vi "meTEC_Re-Init after Error (Monitoring Loop).vi"(8 "error in (no error)":errorcluster) -> (0 "error out":errorcluster)   [LabVIEW 2019]
panel:
  # "--- Outputs ---"
  # "--- Inputs ---"
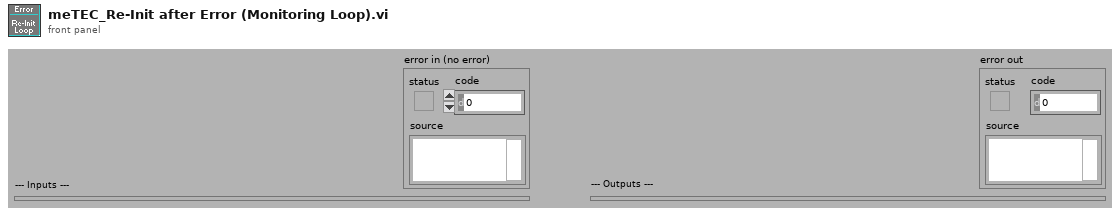
[diagram p1: front panel]
types:
  T1 = typedef "FGV_TE Controller.ctl" = cluster{"SVs":cluster{"Unused":dbl}, "PVs":cluster{"FW & HW Versions":cluster{"Device Type [I32]":i32, "Device Type [String]":string, "Firmware Version [I32]":i32, "Firmware Version [String]":string, "Hardware Version [I32]":i32, "Hardware Version [String]":string, "Serial No.":i32}, "TEC Configuration":T2, "Object Target Temperature Source_CH1":u8, "Object Target Temperature Source_CH2":u8}, "Front Panel References":T3}
  T2 = typedef "meTEC_Configuration.ctl" = cluster{"VISA resource name":refnum<visa-resource-name>, "Device Address":u16}
  T3 = typedef "FGV_Front Panel References.ctl" = cluster{"Main Loop Queue":refnum<queue>, "meTEC_Device Type":refnum<vi>, "meTEC_Serial No.":refnum<vi>, "meTEC_Hardware Version":refnum<vi>, "meTEC_Firmware Version":refnum<vi>, "meTEC_CH1_Object Target Temperature (ID 3000 / 50012) [°C]":refnum<vi>, "meTEC_CH1_Live Set Current (ID 50001) [A]":refnum<vi>, "meTEC_CH1_Live Set Voltage (ID 50002) [V]":refnum<vi>, "meTEC_CH1_Live Enable (ID 50000)":refnum<vi>, "meTEC_CH1_Input Selection (ID 2000)":refnum<vi>, "meTEC_CH1_Object Target Temp. Source Sel. (ID 50011)":refnum<vi>, "meTEC_CH2_Object Target Temperature (ID 3000 / 50012) [°C]":refnum<vi>, "meTEC_CH2_Live Set Current (ID 50001) [A]":refnum<vi>, "meTEC_CH2_Live Set Voltage (ID 50002) [V]":refnum<vi>, "meTEC_CH2_Live Enable (ID 50000)":refnum<vi>, "meTEC_CH2_Input Selection (ID 2000)":refnum<vi>, "meTEC_CH2_Object Target Temp. Source Sel. (ID 50011)":refnum<vi>, "meTEC_CH2_Object Temperature [°C]":refnum<vi>, "meTEC_CH2_Sink Temperature [°C]":refnum<vi>, "meTEC_CH2_Act. Output Current [A]":refnum<vi>, "meTEC_CH2_Act. Output Voltage [V]":refnum<vi>, "meTEC_CH2_Temperature Stability":refnum<vi>, "Monitor Chart_CH2":refnum<vi>, "meTEC_Initialize Device":refnum<vi>}
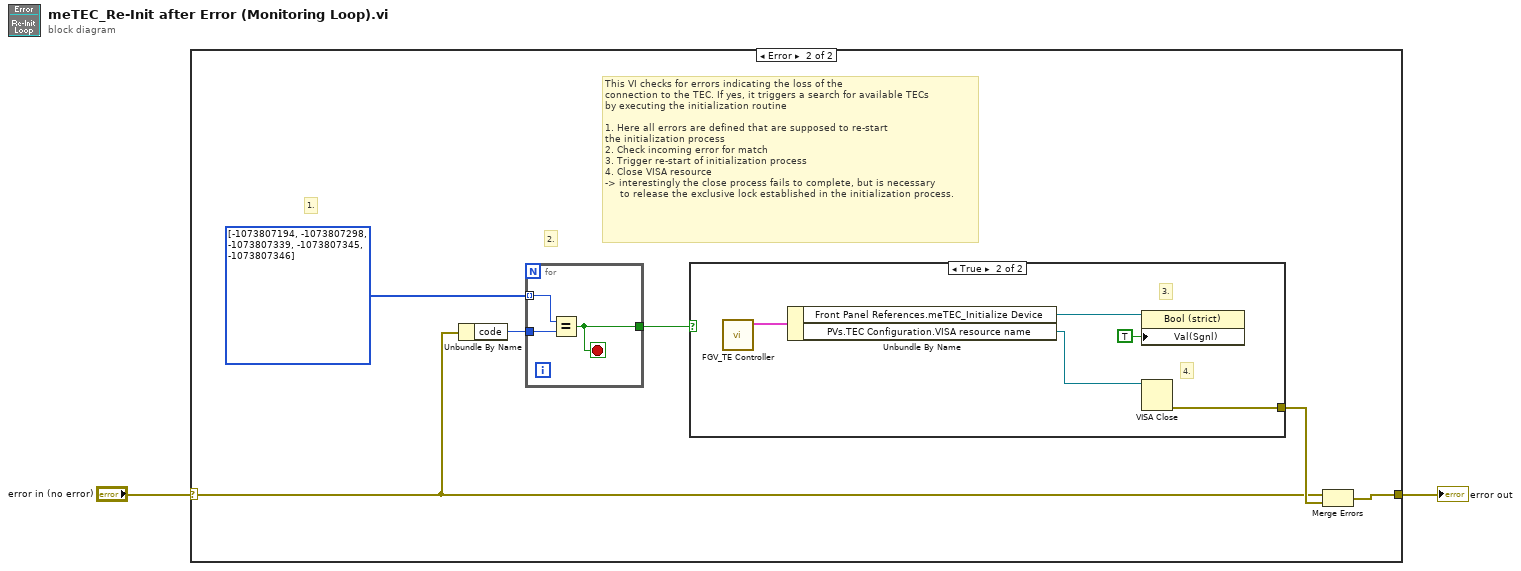
[diagram p0: block diagram]
diagram:
  n1 = case shown="Error" "error in (no error)" {
    selector: "error in (no error)" -> [w3 w5]
    tunnel: [w3 w4] -> w1
    frame No Error {
    }
    frame Error {
      # "This VI checks for errors indicating the loss of the\nconnection to the TEC. If yes, it triggers a search for available TECs\nby executing the initialization routine\n\n1. Here all errors are defined that are supposed to re-start \nthe initialization process\n2. Check incoming error for match\n3. Trigger re-start of initialization process\n4. Close VISA resource\n-> interestingly the close process fails to complete, but is necessary\n     to release the exclusive lock established in the initialization process."
      # "2."
      # "1."
      n2 = Unbundle By Name(w5) -> ("code"=w9:i32)
      n3 = for {
        tunnel: w9 -> [w17]
        tunnel: i32[] [-1073807194, -1073807298, -1073807339, -1073807345, -1073807346] -> [w16] mode=indexing
        tunnel: [w15] -> w7
        stop <- w15 stop-if-true
        n4 = Equal?(x=w16, y=w17) -> (x = y?=w15:bool)
      }
      n5 = case shown="True" w7 {
        tunnel: [_ w11] -> w6
        frame False {
        }
        frame True {
          # "4."
          # "3."
          n6 = call "FGV_TE Controller.vi"() -> ("FGV_TEC_OUT"=w14:T1)  [unwired: 10 in, 1 out]
          n7 = Unbundle By Name(w14) -> ("Front Panel References.meTEC_Initialize Device"=w13:refnum<vi>, "PVs.TEC Configuration.VISA resource name"=w10:refnum<visa-resource-name>)
          n8 = property class="Bool (strict)"(reference=w13, "Val(Sgnl)"=TRUE ("Value (Signaling)")) -> ()  [unwired: 1 in, 2 out]
          n9 = VISA Close(VISA resource name=w10) -> (error out=w11:errorcluster)  [unwired: 1 in]
        }
      }
      n10 = Merge Errors(w5, w6) -> (w4:errorcluster)
    }
  }
  "error out" <- w1
